vi "Shift 2D U32 Array.vi"(8 "error in (no error)":errorcluster caption="错误输入（无错误）", 9 "选择行列":enum16{"行", "列"}(ring), 10 "n":i32, 11 "Input Array":u32[][](array[numeric])) -> (0 "error out":errorcluster caption="错误输出", 3 "Output Array":u32[][](array[numeric]))   [LabVIEW 2012]
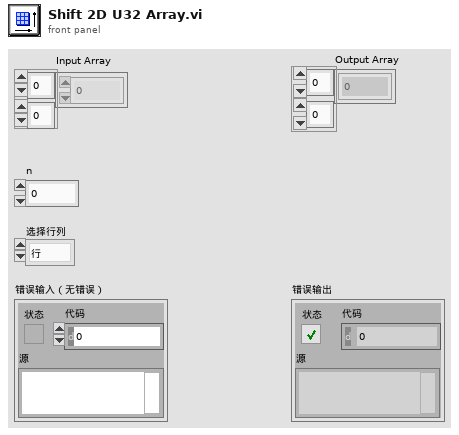
[diagram p1: front panel]
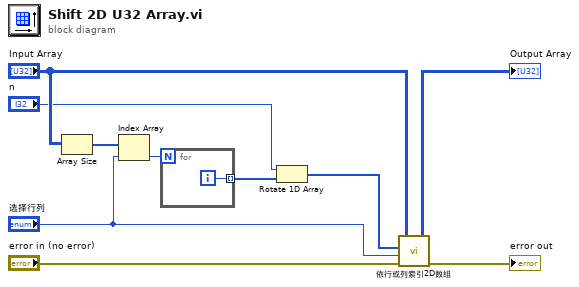
[diagram p0: block diagram]
diagram:
  n1 = Array Size(array="Input Array") -> (size(s)=w6:i32[])
  n2 = Index Array(array=w6, index="选择行列") -> (element=w4:i32)
  n3 = for {
    N: w4 -> [_]
    tunnel: [w11] -> w10 mode=indexing
    i -> [w11]
  }
  n4 = Rotate 1D Array(1:w10, 2:"n") -> (0:w8:i32[])
  n5 = call-poly "依行或列索引2D数组.vi"("error in (no error)"="error in (no error)", "选择行列"="选择行列", "索引"=w8, "输入数组"="Input Array") -> ("error out"=→"error out":errorcluster, "元素"=→"Output Array":u32[][])  [unwired: 6 in]
